vi "chipKIT WF32.vi"() -> (0 "chipKIT WF32":T1={"DI Channels"=[0, 1, 2, 3, 4, 5, 6, 7, 8, 9, 10, 11, 12, 13, 26, 27, 28, 29, 30, 31, 32, 33, 34, 35, 36, 37, 38, 39, 40, 41], "DO Channels"=[0, 1, 2, 3, 4, 5, 6, 7, 8, 9, 10, 11, 12, 13, 26, 27, 28, 29, 30, 31, 32, 33, 34, 35, 36, 37, 38, 39, 40, 41, 43], "AI"=[0, 1, 2, 3, 4, 5, 6, 7, 8, 9, 10, 11], "AO"=[], "PWM"=[3, 5, 6, 9, 10], "QE"=[], "UART"=[0, 1], "I2C 2"=[0], "SPI"=[0], "CAN"=[], "AI Ref (V)"=3.3, "Firmware Program Interfaces"=[enum."Serial / USB"], "Firmware Versions"=[{"Name"="LINX -  Serial / USB", "Relative Path"="\\Digilent\\chipKIT\\WF32\\WF32_Serial_USB.hex", "Firmware Interface"=enum."Serial "}, {"Name"="LINX -  Serial / USB [Debug] ", "Relative Path"="\\Digilent\\chipKIT\\WF32\\WF32_Serial_USB_Debug.hex ", "Firmware Interface"=enum."Serial "}, {"Name"="LINX -  WIFI", "Relative Path"="\\Digilent\\chipKIT\\WF32\\WF32_Wifi.hex ", "Firmware Interface"=enum."WIFI"}, {"Name"="LINX -  WIFI [Debug]", "Relative Path"="\\Digilent\\chipKIT\\WF32\\WF32_Wifi_Debug.hex ", "Firmware Interface"=enum."WIFI"}], "Name"="chipKIT WF32", "AO Resolution (Bits)"=0, "AO Ref (V)"=0.0})   [LabVIEW 2018, in "LVH-LINX.lvlib"]
doc: "I/O description of the chipKIT uC32."
uses:
  LVH-LINX.lvlib
  Generic Device.ctl
  Firmware Version.ctl
  Device/Type Defs/Firmware Interface.ctl
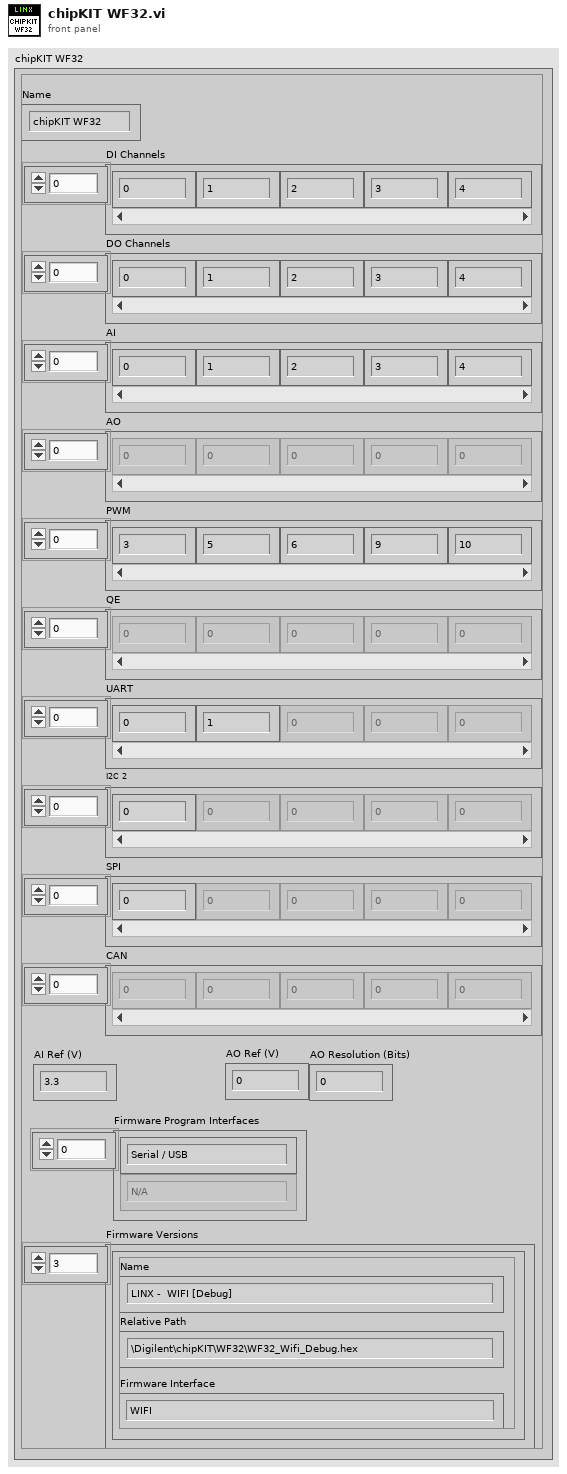
[diagram p1: front panel]
types:
  T1 = typedef "LVH-LINX.lvlib/Generic Device.ctl" = cluster{"DI Channels":u8[], "DO Channels":u8[], "AI":u8[], "AO":u8[], "PWM":u8[], "QE":u8[], "UART":u8[], "I2C 2":u8[], "SPI":u8[], "CAN":u8[], "AI Ref (V)":dbl, "Firmware Program Interfaces":enum16{"N/A", "Serial / USB", "USB", "TCP"}[], "Firmware Versions":T2[], "Name":string, "AO Resolution (Bits)":u8, "AO Ref (V)":dbl}
  T2 = typedef "LVH-LINX.lvlib/Firmware Version.ctl" = cluster{"Name":string, "Relative Path":string, "Firmware Interface":T3}
  T3 = typedef "LVH-LINX.lvlib/Firmware Interface.ctl" = enum32{"Serial ", "Ethernet", "WIFI"}
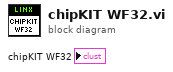
[diagram p0: block diagram]
diagram:
